vi "set current selection (multiple).vi"(8 "error in (no error)":errorcluster, 10 "paths":string[](array[string]), 11 "alias-tree in":refnum<class "alias-tree.lvclass">) -> (0 "error out":errorcluster, 1 "invalid path":bool, 2 "invalid paths":string[](array[string]), 3 "alias-tree out":refnum<class "alias-tree.lvclass">)   [LabVIEW 2017, in "vs-tree-utility.lvlib" / "alias-tree.lvclass"]
uses:
  alias-tree.lvclass
  NationalInstruments.VeriStand.SystemDefinitionAPI
  NationalInstruments.VeriStand.SystemStorageUI
  NationalInstruments.VeriStand.SystemStorage
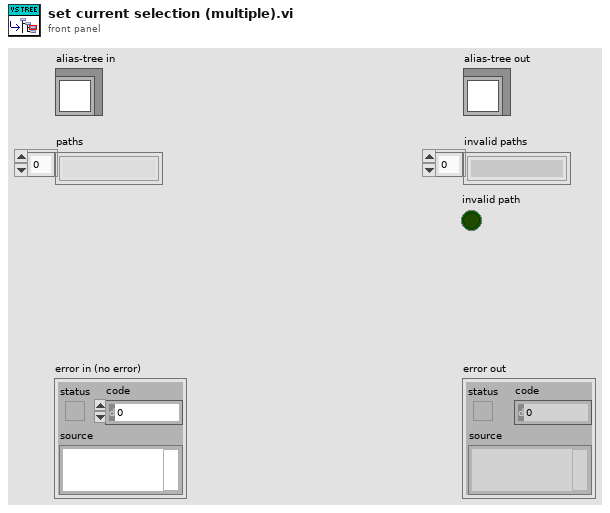
[diagram p1: front panel]
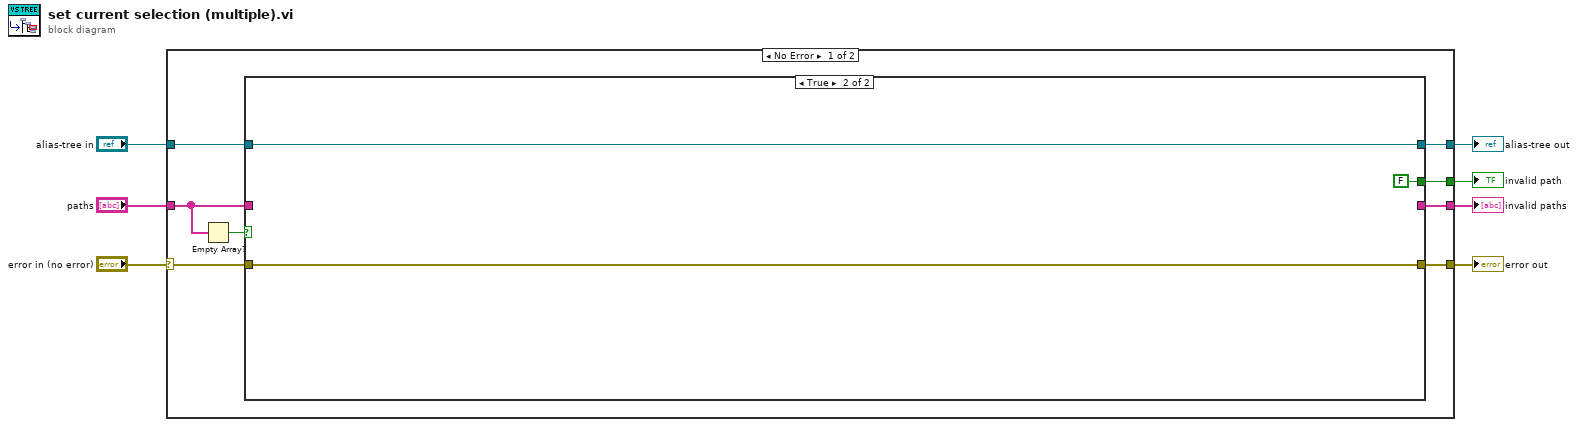
[diagram p0: block diagram]
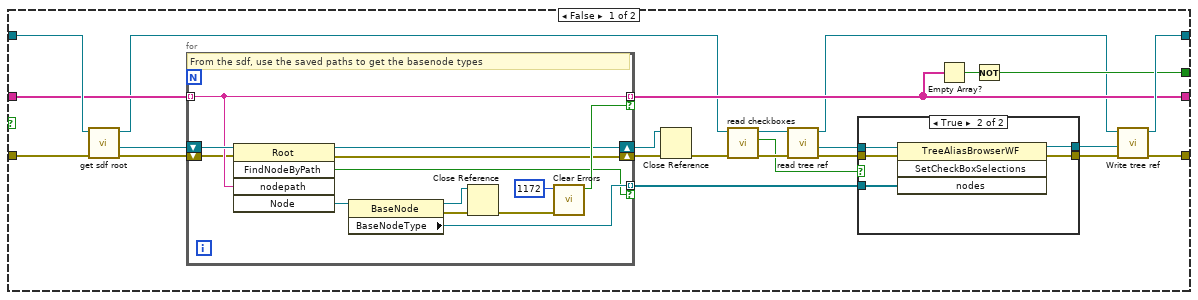
[diagram p2: hidden frame]
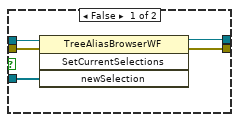
[diagram p3: hidden frame]
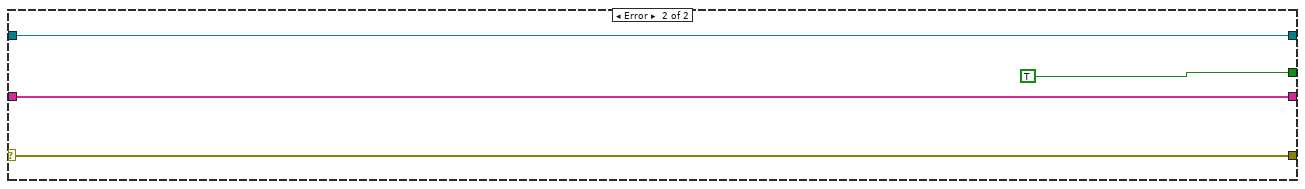
[diagram p4: hidden frame]
diagram:
  n1 = case shown="No Error" "error in (no error)" {
    selector: "error in (no error)" -> [w15 w68]
    tunnel: [w13 w68] -> w6
    tunnel: [w12 w67] -> w5
    tunnel: "alias-tree in" -> [w14 w67]
    tunnel: [w11 w65] -> w3
    tunnel: "paths" -> [w8 w65]
    tunnel: [w10 TRUE] -> w1
    frame No Error {
      n2 = Empty Array?(array=w8) -> (empty?=w9:bool)
      n3 = case shown="True" w9 {
        tunnel: w15 -> [w38 w64]
        tunnel: w14 -> [w37 w62]
        tunnel: w8 -> [w34 _]
        tunnel: [w29 w64] -> w13
        tunnel: [w28 w62] -> w12
        tunnel: [w23 _] -> w11
        tunnel: [w21 FALSE] -> w10
        frame False {
          n4 = call-dynamic "get sdf root.vi"("error in (no error)"=w38, "abstract-tree in"=w37) -> ("error out"=w36:errorcluster, "sdf root"=w35:refnum<k24>, "abstract-tree out"=w19:refnum<class "alias-tree.lvclass">)  [unwired: 7 in]
          n5 = for {
            tunnel: w34 -> [w56] mode=indexing
            tunnel: [w59] -> w25 mode=indexing if=w49
            tunnel: [w56] -> w23 mode=indexing if=w55
            shift-right: [w53] -> w33
            shift-left: w36 -> [w54]
            shift-right: [w52] -> w31
            shift-left: w35 -> [w61]
            # "From the sdf, use the saved paths to get the basenode types"
            n6 = invoke class="Root" method="FindNodeByPath"(reference=w61, error in=w54, "nodepath"=w56) -> (reference out=w52:refnum<k24>, error out=w53:errorcluster, "FindNodeByPath"=w49:bool, "Node"=w60:refnum<k24>)  [unwired: 2 in, 1 out]
            n7 = property class="BaseNode"(reference=w60) -> (reference out=w50:refnum<k24>, error out=w58:errorcluster, "BaseNodeType"=w59:refnum<k24>)  [unwired: 1 in]
            n8 = Close Reference(reference=w50, error in (no error)=w58) -> (error out=w51:errorcluster)
            n9 = call <vilib>:"Clear Errors.vi"("error in (no error)"=w51, "specific error code to clear (0: all)"=1172) -> ("specific error cleared?"=w55:bool)  [unwired: 4 in, 1 out]
          }
          n10 = Close Reference(reference=w31, error in (no error)=w33) -> (error out=w32:errorcluster)
          n11 = call-dynamic "read checkboxes.vi"("error in (no error)"=w32, "alias-tree in"=w19) -> ("error out"=w20:errorcluster, "checkboxes"=w17:bool, "alias-tree out"=w18:refnum<class "alias-tree.lvclass">)  [unwired: 7 in]
          n12 = call-dynamic "read tree ref.vi"("error in (no error)"=w20, "alias-tree in"=w18) -> ("error out"=w30:errorcluster, "tree ref"=w26:refnum<k24>, "alias-tree out"=w16:refnum<class "alias-tree.lvclass">)  [unwired: 7 in]
          n13 = case shown="True" w17 {
            tunnel: w30 -> [w43 w48]
            tunnel: [w42 w45] -> w27
            tunnel: w26 -> [w41 w47]
            tunnel: w25 -> [w40 w46]
            tunnel: [w39 w44] -> w24
            frame False {
              n14 = invoke class="TreeAliasBrowserWF" method="SetCurrentSelections"(reference=w41, error in=w43, "newSelection"=w40) -> (reference out=w39:refnum<k24>, error out=w42:errorcluster)  [unwired: 1 in, 2 out]
            }
            frame True {
              n15 = invoke class="TreeAliasBrowserWF" method="SetCheckBoxSelections"(reference=w47, error in=w48, "nodes"=w46) -> (reference out=w44:refnum<k24>, error out=w45:errorcluster)  [unwired: 1 in, 2 out]
            }
          }
          n16 = Empty Array?(array=w23) -> (empty?=w22:bool)
          n17 = Not(x=w22) -> (.not. x?=w21:bool)
          n18 = call-dynamic "Write tree ref.vi"("error in (no error)"=w27, "tree ref"=w24, "alias-tree in"=w16) -> ("error out"=w29:errorcluster, "alias-tree out"=w28:refnum<class "alias-tree.lvclass">)  [unwired: 7 in]
        }
        frame True {
        }
      }
    }
    frame Error {
    }
  }
  "error out" <- w6
  "alias-tree out" <- w5
  "invalid paths" <- w3
  "invalid path" <- w1
